vi "MM9.PG_getConfigKnorz.vi"(0 "i ref in":refnum<vi>, 5 "error in (no error)":errorcluster) -> (14 "i ref out":refnum<vi>, 16 "PGData":T1, 19 "error out":errorcluster)   [LabVIEW 2014, in "MM9.lvlib"]
doc: "This is real \"Knorz\". Try to get the trigger stuff from the database (via the BaseProcess attribute), analyze the attribute data of this class to get the \"memory\" configuration.\n\nFirst, a better solution would be to obtain the trigger conditions not via the database but via user input. \nSecond, the number of the actual configuration (for a \"switch measurement\") needs to be implemented."
uses:
  MM9.lvlib
  CSDigitalIO/PPG_ABC/PPG_ABC.PG_dataType.ctl
  CSCore/BaseProcess/BaseProcess.lvlib
  LEBITLib/LEBITLib.lvlib
  CSDigitalIO/PPG_ABC/PPG_ABC.lvlib
panel:
  in  "PGDataType":T1
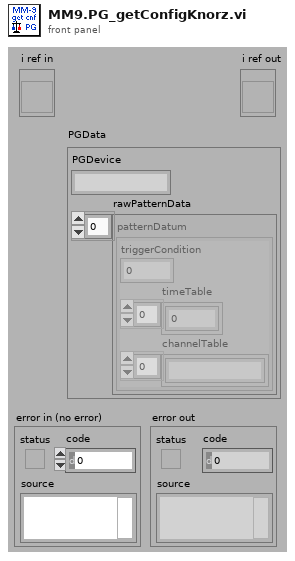
[diagram p1: front panel]
types:
  T1 = typedef "PPG_ABC.lvlib/PPG_ABC.PG_dataType.ctl" = cluster{"PGDevice":string, "rawPatternData":cluster{"triggerCondition":i32, "timeTable":dbl[], "channelTable":string[]}[]}
  T2 = typedef "BaseProcess.lvlib/BaseProcess.i attribute.ctl" = cluster{"EventStatus":string, "EventError":i32, "PresetEvtWatchD":i32, "PresetPdcWatchD":i32, "EventTimeout":i32, "PeriodicInterval":i32, "Interface":string[], "Address":string[], "Special":string[], "PeriodicError":i32, "PeriodicStatus":string, "SuperProc":string, "Descriptors":T3[], "CaseRef":refnum<vi>, "PdcRef":refnum<vi>, "Thread Ref":refnum<vi>, "eventErrorID":i32, "eventStatusID":i32, "periodicErrorID":i32, "periodicStatusID":i32, "pdcCtrID":i32}
  T3 = typedef "BaseProcess.lvlib/BaseProcess.descriptor definition.ctl" = cluster{"selector":string, "descriptor":T4}
  T4 = typedef "BaseProcess.lvlib/BaseProcess.descriptor string definition.ctl" = string
  T5 = typedef "MM9.lvlib/MM9.i attribute.ctl" = cluster{"UsedObjs":string[], "ActScanStep":i32[], "AbortRequest":bool, "StopRequest":bool, "# cycles":i32, "Connected":bool, "MMStatus":T6, "# data":i32, "DIMServices":cluster{"MM6StatusString":string, "MM6StatusID":i32, "discArchiver":string, "discArchiverID":i32, "eventBuilder":string, "eventBuilderID":i32, "GUIIDString":string, "GUIIDStringID":i32}, "dataFile":string, "PGRunning":T7, "ConfigData":T8, "ExtraDataSets":T23}
  T6 = typedef "MM9.lvlib/MM9.status.ctl" = enum16{"loaded", "load_error", "config", "config_error", "init", "init_error", "data_reset", "data_reset_error", "running", "start_error", "run_error", "abort_requested", "aborted", "stop_requested", "stopped", "stop_error", "Connected", "NOTConnected"}
  T7 = typedef "PPG_ABC.lvlib/PPG_ABC.PG_Running.ctl" = i32
  T8 = typedef "LEBITDefs9.lvlib/LEBITDefs.ConfigData.ctl" = cluster{"GenConfig":T9, "Configs":T11[]}
  T9 = typedef "LEBITDefs9.lvlib/LEBITDefs.GenConfig.ctl" = cluster{"Mode":i32, "Logs":T10[]}
  T10 = typedef "LEBITDefs9.lvlib/LEBITDefs.Log.ctl" = cluster{"Name":string, "FctName":string, "Special":string}
  T11 = typedef "LEBITDefs9.lvlib/LEBITDefs.OneConfig.ctl" = cluster{"MCA":T12, "Timing":T13, "Scans":T16[], "FreqDevs":T17[], "CleanDev":T18, "NrCycles":i32, "Specials":T20[], "Delays":T21[], "DAC":T22}
  T12 = typedef "LEBITDefs9.lvlib/LEBITDefs.MCA.ctl" = cluster{"Name":string, "Address":string, "NrChannels":i32, "Gate":i32, "NrPipse":i32, "AcqDelay":i32}
  T13 = typedef "LEBITDefs9.lvlib/LEBITDefs.Timing.ctl" = cluster{"TimeTables":cluster{"TimeTable":T14}[], "Memories":T15[], "ScanX":string, "ScanY":string}
  T14 = typedef "LEBITDefs9.lvlib/LEBITDefs.Timetable.ctl" = dbl[]
  T15 = typedef "LEBITDefs9.lvlib/LEBITDefs.Memory.ctl" = cluster{"Device":string, "ExtTrig":bool, "TT2Use":i32, "PatternTable":string[]}
  T16 = typedef "LEBITDefs9.lvlib/LEBITDefs.ScanDev.ctl" = cluster{"Name":string, "FctName":string, "Values":dbl[], "NrScanVals":i32, "Special":string}
  T17 = typedef "LEBITDefs9.lvlib/LEBITDefs.FreqDev.ctl" = cluster{"Name":string, "Amp":dbl, "CenterFreq":dbl, "Time":dbl}
  T18 = typedef "LEBITDefs9.lvlib/LEBITDefs.CleanDev.ctl" = cluster{"Name":string, "CleanData":T19[]}
  T19 = typedef "LEBITDefs9.lvlib/LEBITDefs.CleanDataType.ctl" = cluster{"Amp":dbl, "Center":dbl, "Plus":dbl, "Minus":dbl, "Time":dbl}
  T20 = typedef "LEBITDefs9.lvlib/LEBITDefs.Special.ctl" = cluster{"Name":string, "FctName":string, "VerySpecial":string, "Data":dbl}
  T21 = typedef "LEBITDefs9.lvlib/LEBITDefs.Delay.ctl" = cluster{"Name":string, "Delay":dbl}
  T22 = typedef "LEBITDefs9.lvlib/LEBITDefs.DAC.ctl" = cluster{"Name":string, "Step1":i32, "Step2":i32}
  T23 = typedef "LEBITDefs9.lvlib/LEBITDefs.ExtraData.ctl" = cluster{"Ions":cluster{"ExcitIonMass":string, "ExcitIonCharge":i32, "CleanIons":cluster{"CleanIonMass":string, "CleanIonCharge":i32}[]}, "TimingDescription":cluster{"TimeTableDescription":cluster{"Times":string[]}[], "PatternTableDescription":cluster{"Pattern":string[]}[]}, "ScanUnits":string[]}[]
  T24 = cluster{"triggerCondition":i32, "timeTable":dbl[], "channelTable":string[]}[]
  T25 = cluster{"triggerCondition":i32, "timeTable":dbl[], "channelTable":string[]}
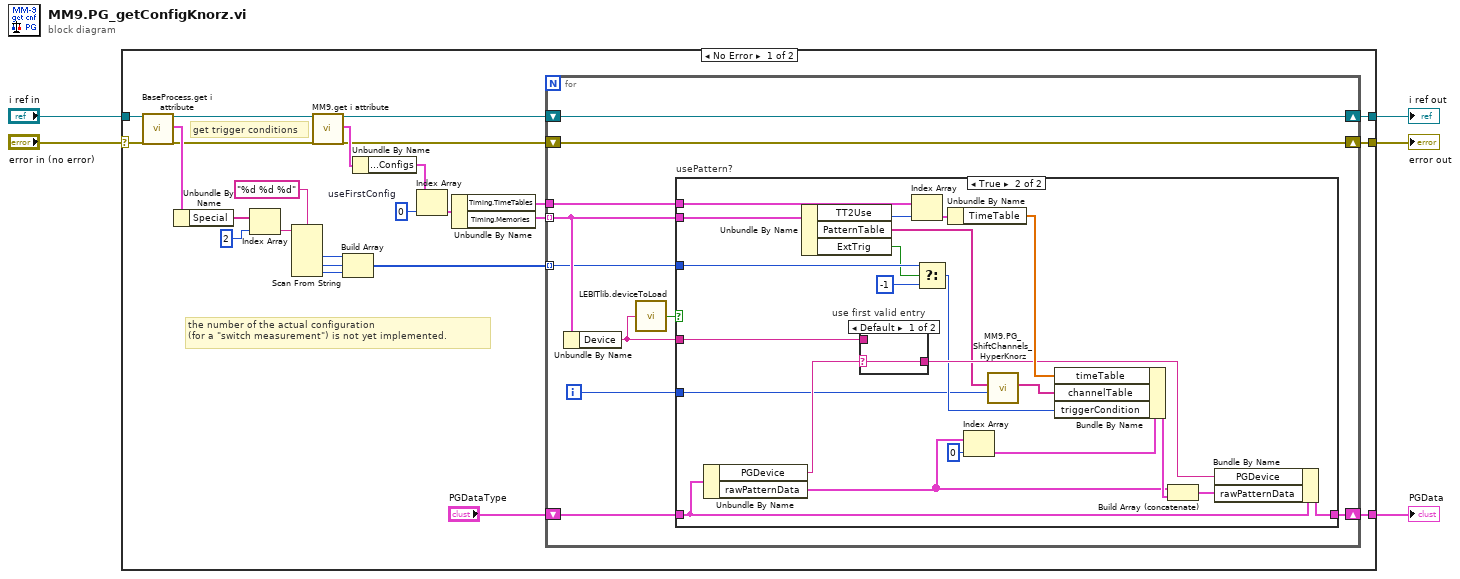
[diagram p0: block diagram]
diagram:
  n1 = case shown="No Error" "error in (no error)" {
    selector: "error in (no error)" -> [w26 w66]
    tunnel: "i ref in" -> [w30 w67]
    tunnel: [w15 w67] -> w4
    tunnel: [w14 w66] -> w3
    tunnel: [w6 _] -> w1
    frame No Error {
      w19 = 0  # useFirstConfig
      # "the number of the actual configuration \n(for a \"switch measurement\") is not yet implemented."
      # "get trigger conditions"
      n2 = call "BaseProcess.get i attribute.vi"("i ref in"=w30, "error in (no error)"=w26) -> ("i ref out"=w21:refnum<vi>, "i attribute"=w29:T2, "error out"=w22:errorcluster)  [unwired: 15 in]
      n3 = Unbundle By Name(w29) -> ("Special"=w28:string[])
      n4 = Index Array(array=w28, index=2) -> (element=w25:string)
      n5 = Scan From String(format string="%d %d %d", input string=w25) -> (output 1=w10:i32, output 2=w9:i32, output 3=w8:i32)  [unwired: 5 in, 3 out]
      n6 = call "MM9.get i attribute.vi"("i ref in"=w21, "error in (no error)"=w22) -> ("i ref out"=w17:refnum<vi>, "i attribute"=w23:T5, "error out"=w16:errorcluster)  [unwired: 15 in]
      n7 = Build Array(w10, w9, w8) -> (w7:i32[])
      n8 = Unbundle By Name(w23) -> ("ConfigData.Configs"=w20:T11[])
      n9 = Index Array(array=w20, index=w19) -> (element=w18:T11)
      n10 = Unbundle By Name(w18) -> ("Timing.TimeTables"=w12:cluster{"TimeTable":T14}[], "Timing.Memories"=w11:T15[])
      n11 = for {
        shift-right: [w33] -> w15
        shift-left: w17 -> [w33]
        shift-right: [w32] -> w14
        shift-left: w16 -> [w32]
        shift-right: [w34] -> w6
        shift-left: "PGDataType" -> [w35]
        tunnel: w12 -> [w38]
        tunnel: w11 -> [w37] mode=indexing
        tunnel: w7 -> [w36] mode=indexing
        i -> [w31]
        n12 = Unbundle By Name(w37) -> ("Device"=w39:string)
        n13 = call "LEBITlib.deviceToLoad.vi"("DeviceName"=w39) -> ("DeviceIsToLoad"=w40:bool)
        n14 = case "usePattern?" shown="True" w40 {
          tunnel: w37 -> [_ w60]
          tunnel: w39 -> [_ w61]
          tunnel: w38 -> [_ w59]
          tunnel: w36 -> [_ w48]
          tunnel: w35 -> [w41 w51]
          tunnel: [w41 w49] -> w34
          tunnel: w31 -> [_ w42]
          frame False {
          }
          frame True {
            n15 = Unbundle By Name(w51) -> ("PGDevice"=w53:string, "rawPatternData"=w54:T24)
            n16 = Unbundle By Name(w60) -> ("TT2Use"=w58:i32, "PatternTable"=w44:string[], "ExtTrig"=w47:bool)
            n17 = case "use first valid entry" shown="Default" w53 {
              selector: w53 -> [w64 _]
              tunnel: w61 -> [_ w65]
              tunnel: [w64 w65] -> w50
              frame Default {
              }
              frame "" {
              }
            }
            n18 = Index Array(array=w59, index=w58) -> (element=w57:cluster{"TimeTable":T14})
            n19 = Select(t=w48, s=w47, f=-1) -> (s? t:f=w45:i32)
            n20 = Unbundle By Name(w57) -> ("TimeTable"=w56:T14)
            n21 = Index Array(array=w54, index=0) -> (element=w62:T25)
            n22 = call "MM9.PG_ShiftChannels_HyperKnorz.vi"("patternNumber"=w42, "PatternTable"=w44) -> ("PatternTableShifted"=w43:string[])  [unwired: 9 in]
            n23 = Bundle By Name(cluster=w62, "timeTable"=w56, "channelTable"=w43, "triggerCondition"=w45) -> (w55:T25)
            n24 = Build Array (concatenate)(w54, w55) -> (w52:T24)
            n25 = Bundle By Name(cluster=w51, "PGDevice"=w50, "rawPatternData"=w52) -> (w49:T1)
          }
        }
      }
    }
    frame Error {
    }
  }
  "error out" <- w3
  "i ref out" <- w4
  "PGData" <- w1
